vi "_FPGA_LUT_of_Cosine_B.vi"(10 "Cycle_in":u16, 11 "NorAmp*2^31":u32) -> (2 "cos":fxp<+,14,14>, 5 "Cross_zero?":bool)   [LabVIEW 2018]
uses:
  <vilib>/rvi/Memory/Memory_Emulation/nirvimemoryFastEmulation.vi
  <vilib>/rvi/Memory/Memory_Emulation/nirvimemoryEmulation.vi
  <vilib>/rvi/Emulation/niFpgaEmulationIsFPGAContextNoSignature.vi
  <vilib>/rvi/DataTransferAndStorage/Container/Common/niFpgaContainerGetUniqueNameForEmu.vi
  <vilib>/rvi/Emulation/niFpgaProcessEmulError.vi
  <vilib>/rvi/Emulation/niFpgaSctlEmulationGetInTimedLoop.vi
  <vilib>/rvi/errors/nirviReportUnexpectedCaseInternalError (U32).vi
  <vilib>/rvi/DataTransferAndStorage/Container/XNode/niFpgaContainer.xnode
  <instrlib>/_niInstr/Basic Elements/v1/FPGA/niInstr Basic Elements v1 FPGA.lvlib
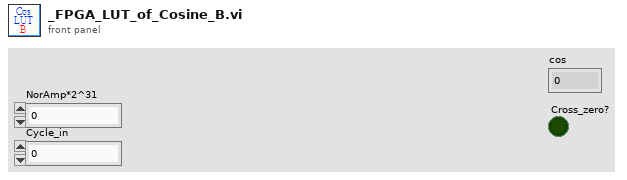
[diagram p1: front panel]
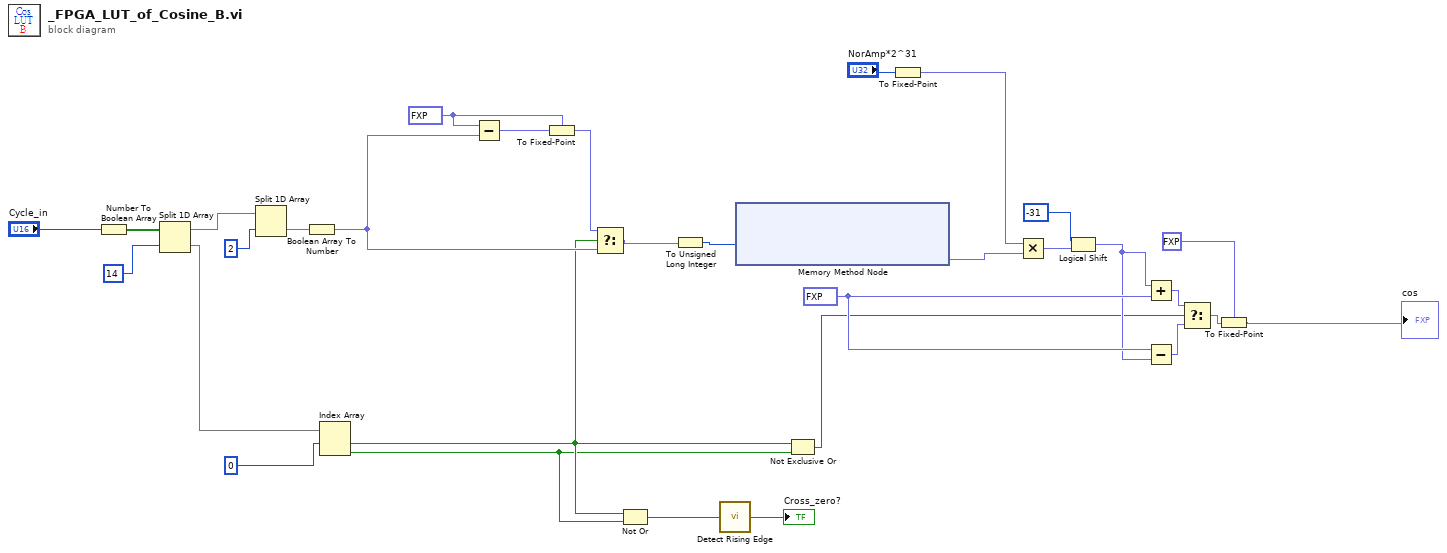
[diagram p0: block diagram]
diagram:
  w22 = fxp<+,13,13> 8191.0
  w23 = fxp<+,14,14> 8192.0
  n1 = Number To Boolean Array(number="Cycle_in") -> (Boolean array=w30:bool[])
  n2 = Split 1D Array(array=w30, index=14) -> (first subarray=w16:bool[], second subarray=w24:bool[])
  n3 = Split 1D Array(array=w16, index=2) -> (second subarray=w15:bool[])  [unwired: 1 out]
  n4 = Boolean Array To Number(Boolean array=w15) -> (number=w18:fxp<+,13,13>)
  n5 = Index Array(array=w24, index #1=0 ("index")) -> (element #1=w5:bool, element #2=w4:bool)  [unwired: 1 in]
  n6 = Subtract(x=w22, y=w18) -> (x-y=w21:fxp<+/-,14,14>)
  n7 = To Fixed-Point(fixed-point type=w22, number=w21) -> (fixed-point=w20:fxp<+,13,13>)
  n8 = Select(t=w20, s=w5, f=w18) -> (s? t:f=w19:fxp<+,13,13>)
  n9 = Not Or(1:w4, 2:w5) -> (0:w1:bool)
  n10 = To Unsigned Long Integer(number=w19) -> (unsigned 32bit integer=w7:u32)
  n11 = call <instrlib>:"Detect Rising Edge.vi"("signal"=w1) -> ("edge detected"=→"Cross_zero?":bool)  [unwired: 14 in]
  n12 = xnode ("Memory Method Node")("Address B"=w7) -> ("Data B"=w6:fxp<+,13,13>)  [unwired: 1 in, 1 out]
  n13 = Not Exclusive Or(1:w4, 2:w5) -> (0:w3:bool)
  n14 = To Fixed-Point(number="NorAmp*2^31") -> (fixed-point=w11:fxp<+,32,32>)  [unwired: 1 in]
  n15 = Multiply(x=w11, y=w6) -> (x*y=w13:fxp<+,45,45>)
  n16 = Logical Shift(y=i16 -31, x=w13) -> (x << y=w9:fxp<+,45,45>)
  n17 = Add(x=w9, y=w23) -> (x+y=w26:fxp<+,46,46>)
  n18 = Subtract(x=w23, y=w9) -> (x-y=w25:fxp<+/-,46,46>)
  n19 = Select(t=w26, s=w3, f=w25) -> (s? t:f=w27:fxp<+/-,47,47>)
  n20 = To Fixed-Point(fixed-point type=fxp<+,14,14> 0.0 ("sine"), number=w27) -> (fixed-point=→"cos":fxp<+,14,14>)
